vi "Suma.vi"(8 "error in (no error)":errorcluster, 11 "VISA resource name":refnum<visa-resource-name>) -> (0 "error out":errorcluster, 3 "VISA resource name 2":refnum<visa-resource-name>)   [LabVIEW 2019, in "Libreria SUBVI´s.lvlib"]
panel:
  out "read buffer":string
  in  "stop":bool
  out "Numeric 3":dbl
  in  "Numeric 2":dbl
  in  "Numeric":dbl
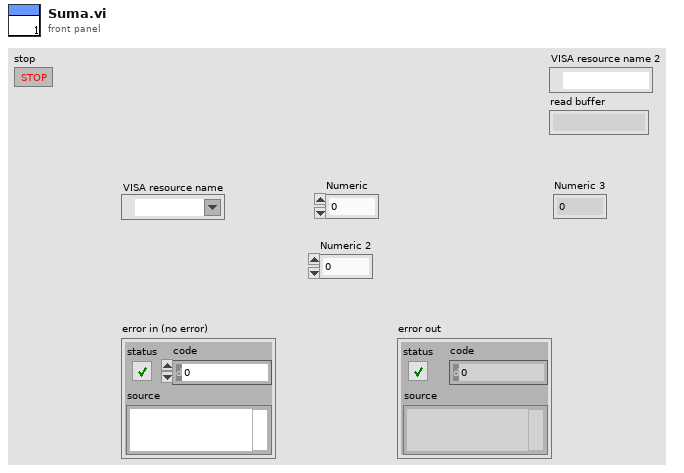
[diagram p1: front panel]
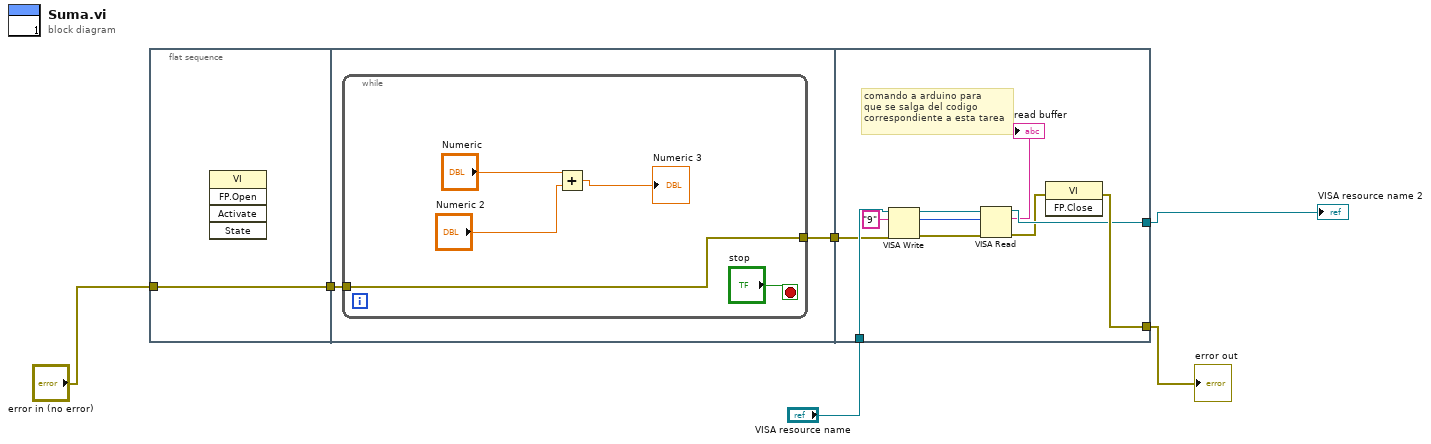
[diagram p0: block diagram]
diagram:
  n1 = flat-sequence {
    tunnel: "error in (no error)" -> [w7]
    tunnel: [w7] -> w2
    tunnel: w2 -> [w9]
    tunnel: [w8] -> w1
    tunnel: [w22] -> w6
    tunnel: "VISA resource name" -> [w24]
    tunnel: [w19] -> w4
    tunnel: w1 -> [w15]
    frame #0 {
      n2 = invoke class="VI" method="FP.Open"() -> ()  [unwired: 5 in, 5 out]
    }
    frame #1 {
      n3 = while {
        tunnel: w9 -> [w10]
        tunnel: [w10] -> w8
        stop <- "stop" stop-if-true
        n4 = Add(x="Numeric", y="Numeric 2") -> (x+y=→"Numeric 3":dbl)
      }
    }
    frame #2 {
      # "comando a arduino para\nque se salga del codigo\ncorrespondiente a esta tarea"
      n5 = VISA Write(VISA resource name=w24, write buffer="9", error in (no error)=w15) -> (VISA resource name out=w21:refnum<visa-resource-name>, return count=w20:u32, error out=w17:errorcluster)
      n6 = VISA Read(VISA resource name=w21, byte count=w20, error in (no error)=w17) -> (VISA resource name out=w19:refnum<visa-resource-name>, read buffer=→"read buffer":string, error out=w16:errorcluster)  [unwired: 1 out]
      n7 = invoke class="VI" method="FP.Close"(error in=w16) -> (error out=w22:errorcluster)  [unwired: 2 in, 2 out]
    }
  }
  "error out" <- w6
  "VISA resource name 2" <- w4
